vi "Measurement UI.vi"() -> ()   [LabVIEW 2021, in "audio_acMeasurement.lvlib"]
uses:
  audio_acMeasurement.lvlib
panel:
  in  "MeasGraphs":T1(tab)
  out "FreqDomainGraph":cluster{"x0":dbl, "dx":dbl, "magnitude":dbl[]}(graph) caption="AC"
  out "TimeDomainGraph":waveform(dbl)(graph) caption="AC"
  in  "JSON file":string
  out "Channel":string
  out "Spectrum":dbl[](array[numeric])
  out "df":dbl
  out "f0":dbl
  out "Time domain":dbl[](array[numeric])
  out "dt":dbl
  out "THD+N":dbl
  out "THD":dbl
  out "SNR":dbl
  out "Calculated amplitude":dbl
  out "Calculated frequency":dbl
  out "SFDR":dbl
  out "Dynamic range":dbl
  out "Gain error":dbl
  in  "Analog source resource name":string
  out "MeasTable":string[][](table)
  in  "File name":string(combo) caption="FILE NAME"
  out "Sample rate":u32 caption="SAMPLE RATE" format="%#.6pHz"
  in  "Protocol capture channel":string="0L" caption="CHANNEL"
  in  "Protocol capture resource name":string caption="RESOURCE NAME"
  in  "Protocol settings":string="Protocol settings"
  in  "Analog source":string="Analog source "
  in  "Full scale range":dbl=3.16 caption="FULL SCALE RANGE" format="%.3pV"
  in  "Measurement settings":string="Measurement settings"
  in  "MeasSettingsOptions":i32(listbox)=-1
  in  "MeasSettings":bool
  in  "DSGResourceName":tag caption="RESOURCE NAME"
  in  "Weighting filter":T2(ring) caption="WEIGHTING FILTER"
  in  "Number of words":u32=19200 caption="NUMBER OF WORDS"
  in  "Clock rate":u32=12288000 caption="CLOCK RATE" format="%#.6pHz"
  in  "Band stop":dbl=20000.0 caption="BAND STOP" format="%#_6pHz"
  in  "Band start":dbl=20.0 caption="BAND START" format="%#_6pHz"
  in  "Amplitude":dbl=-1.0 caption="AMPLITUDE" format="%#_6pdB"
  in  "Frequency":dbl=1000.0 caption="FREQUENCY" format="%#_6pHz"
  in  "Sensitivity":dbl=0.34762 caption="SENSITIVITY" format="%.5fFS/Pa"
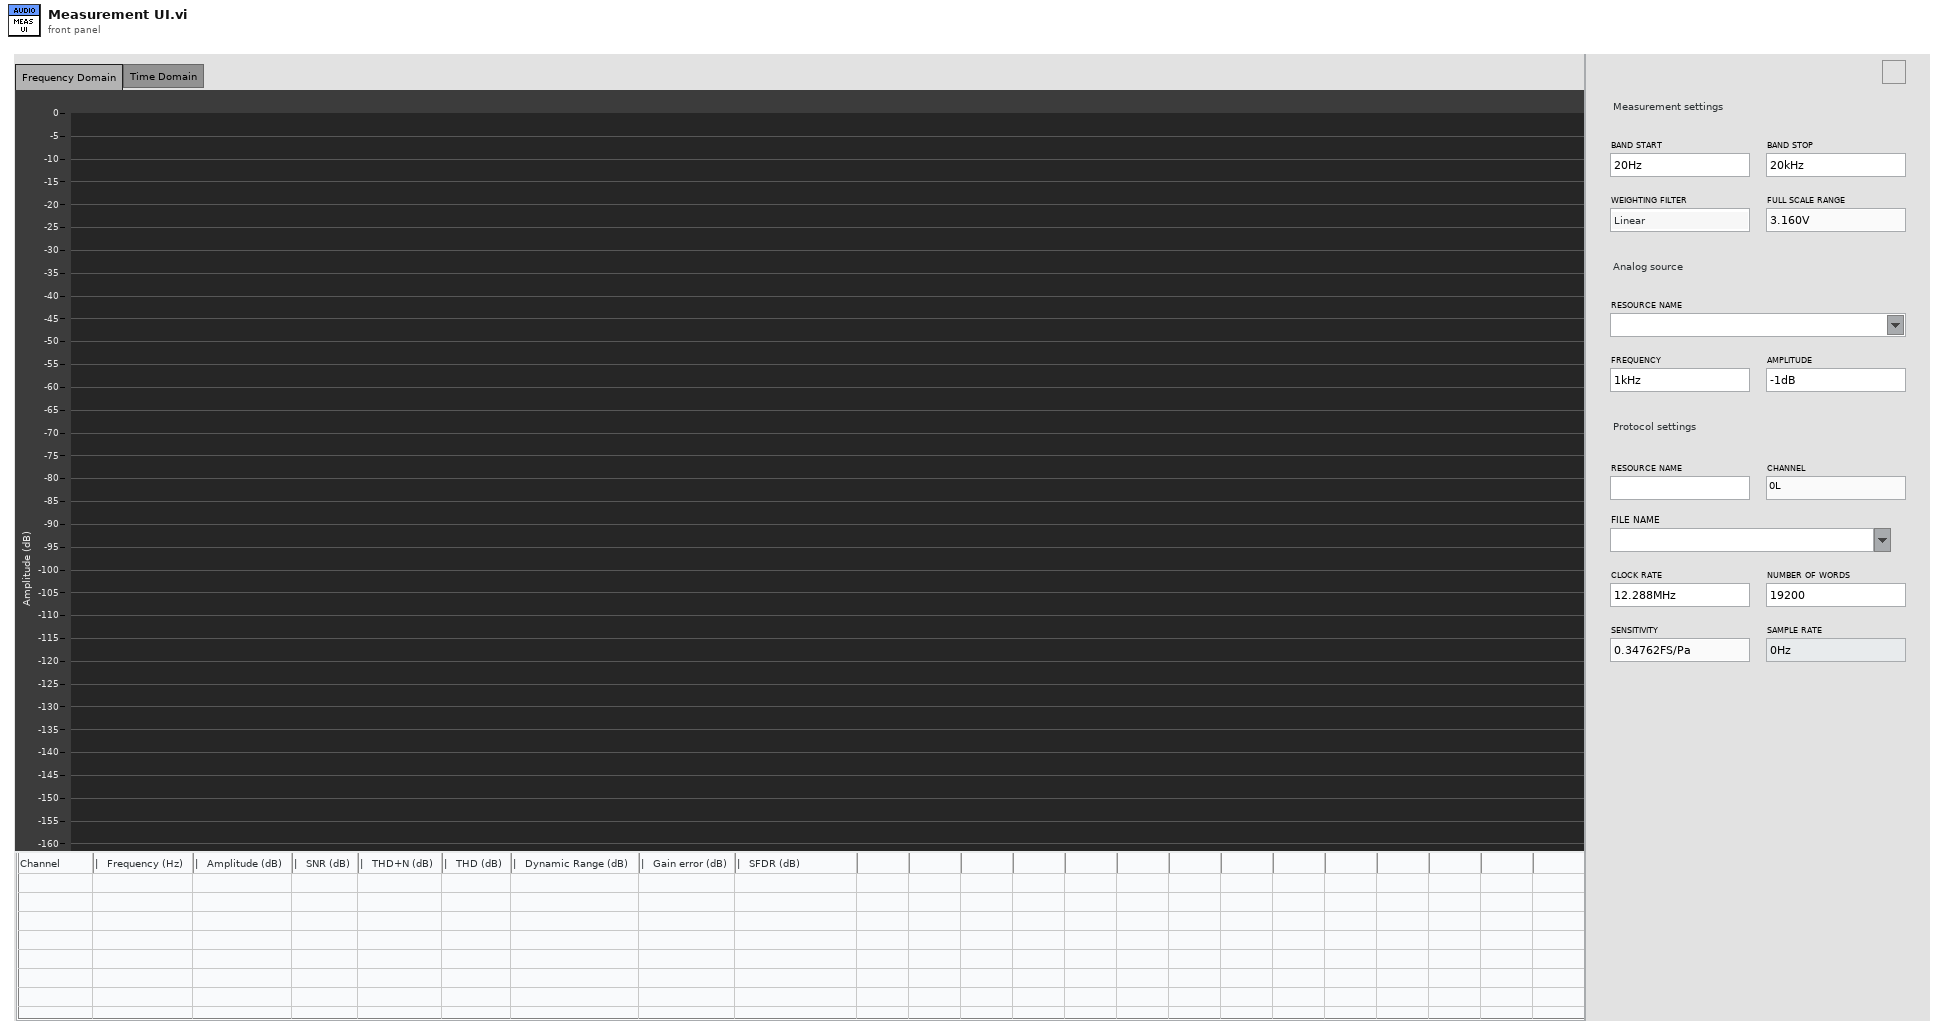
[diagram p1: front panel]
types:
  T1 = enum32{"Frequency Domain", "Time Domain", "Hidden Controls"}
  T2 = enum16{"Linear", "A-Weighting", "B-Weighting", "C-Weighting"}
  T3 = enum16{"open", "replace", "create", "open or create", "replace or create", "replace or create with confirmation"}
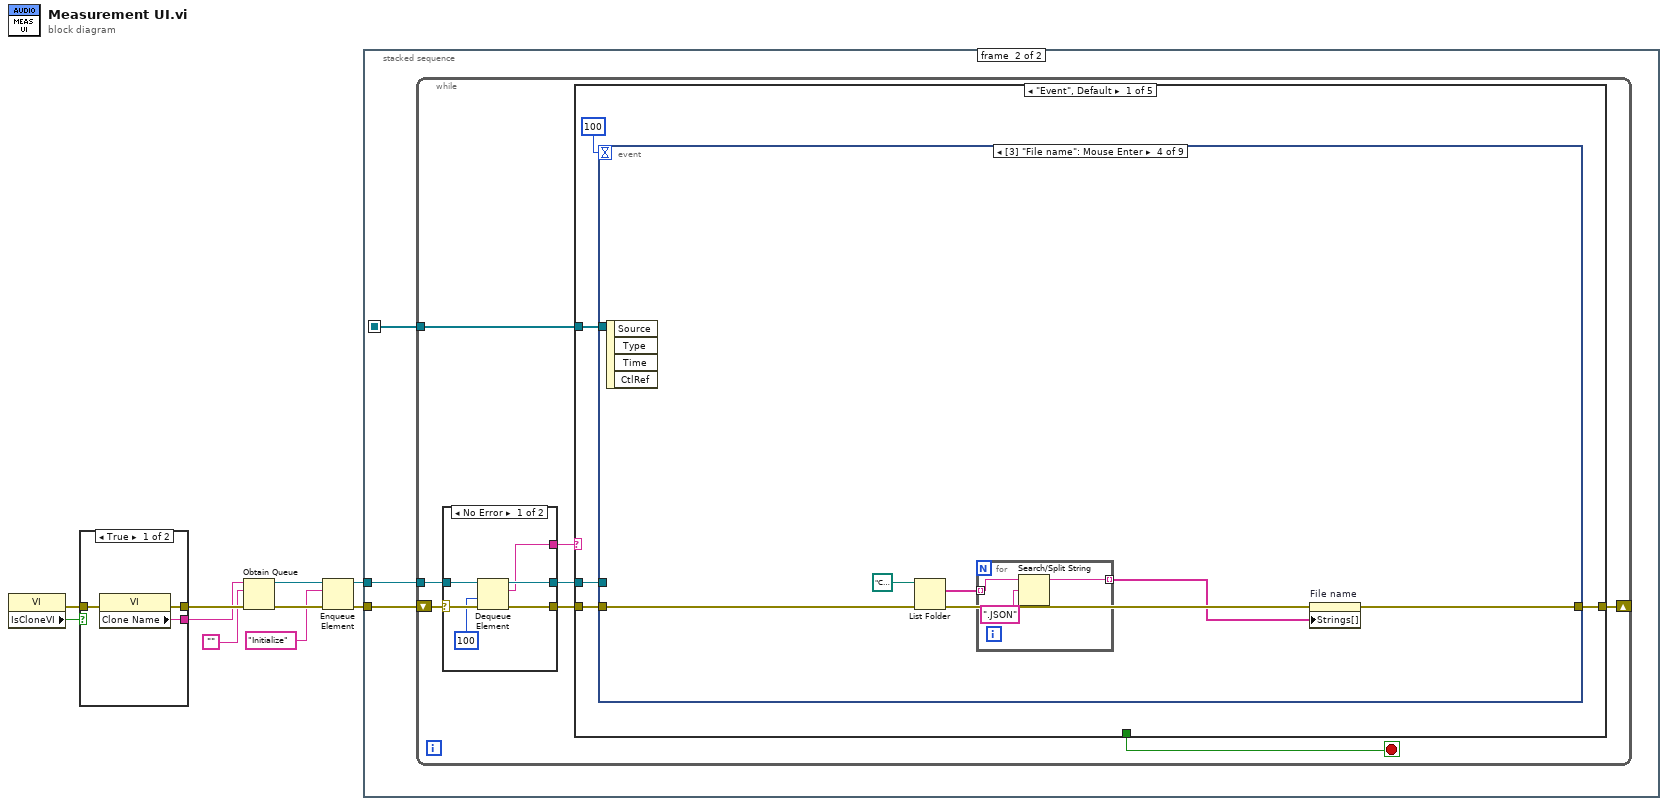
[diagram p0: block diagram]
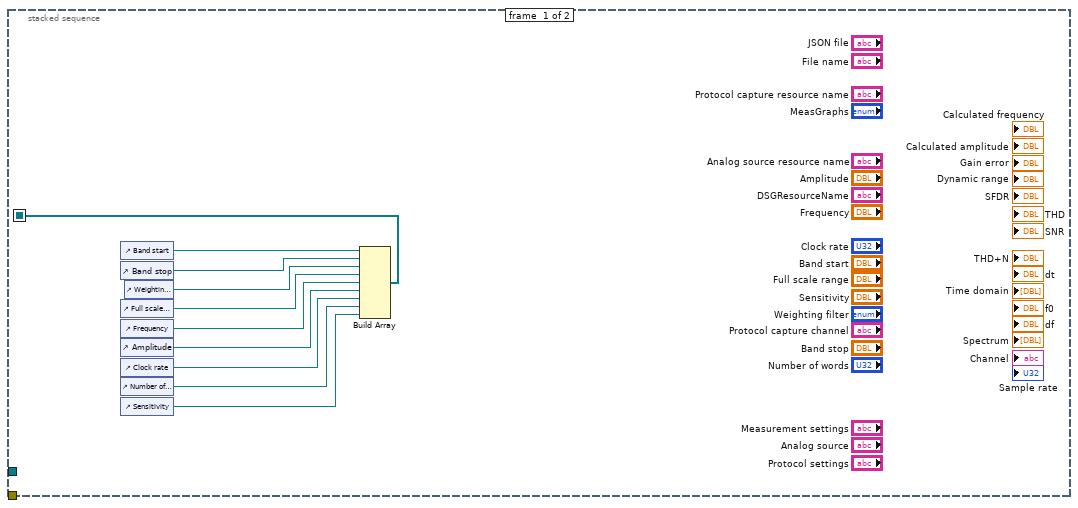
[diagram p2: hidden frame]
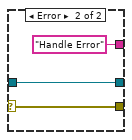
[diagram p3: hidden frame]
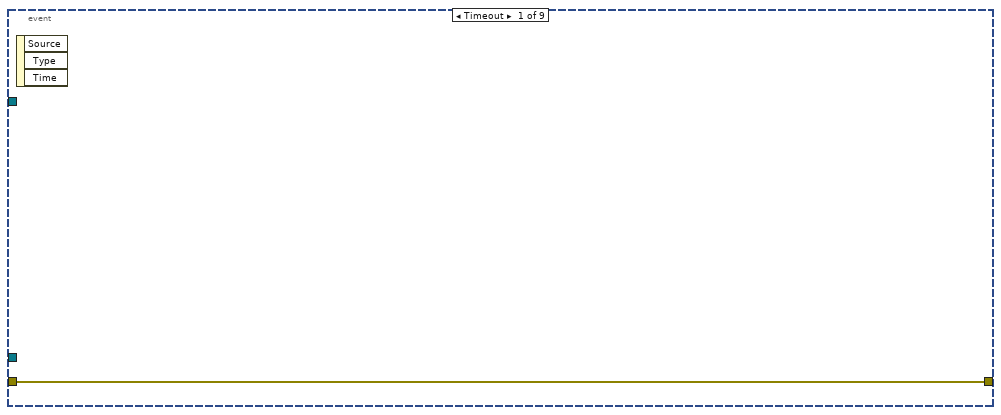
[diagram p4: hidden frame]
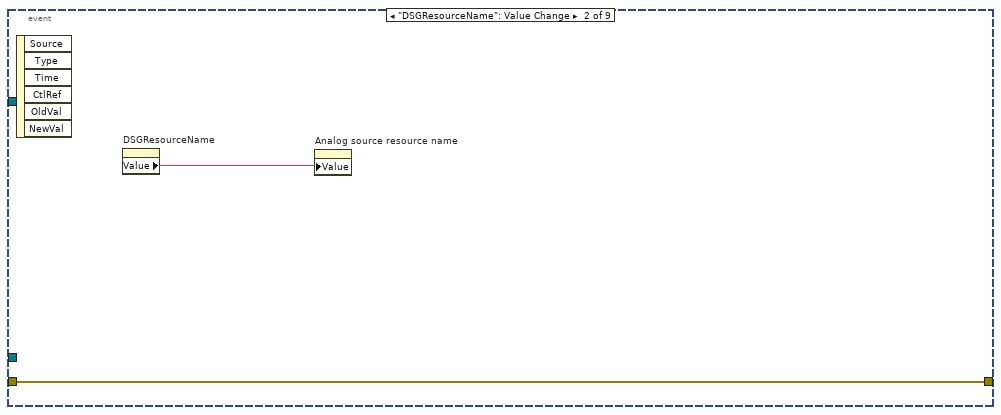
[diagram p5: hidden frame]
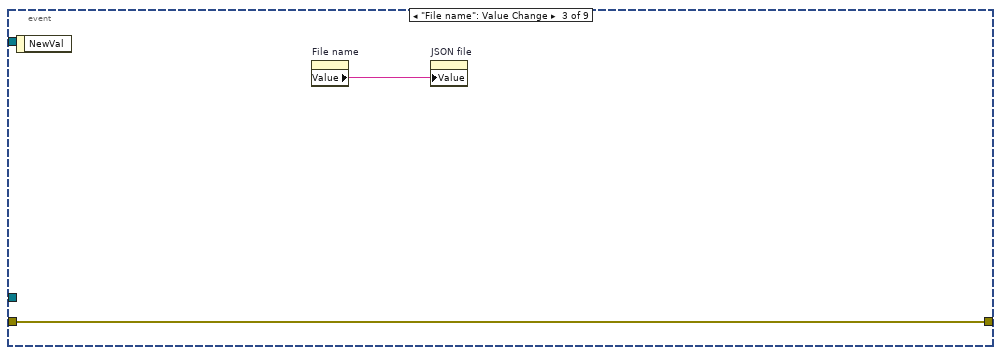
[diagram p6: hidden frame]
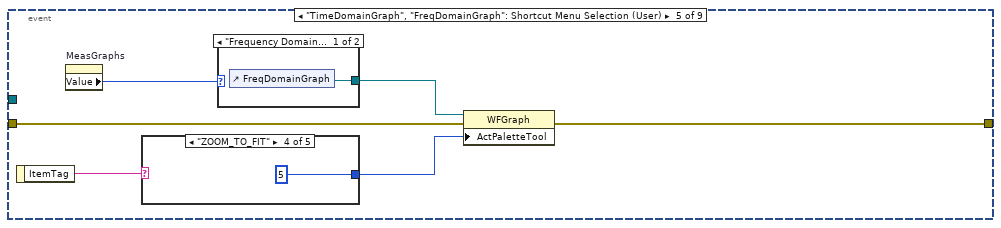
[diagram p7: hidden frame]
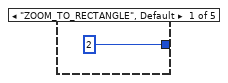
[diagram p8: hidden frame]
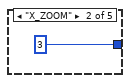
[diagram p9: hidden frame]
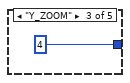
[diagram p10: hidden frame]
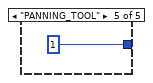
[diagram p11: hidden frame]
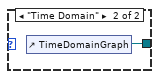
[diagram p12: hidden frame]
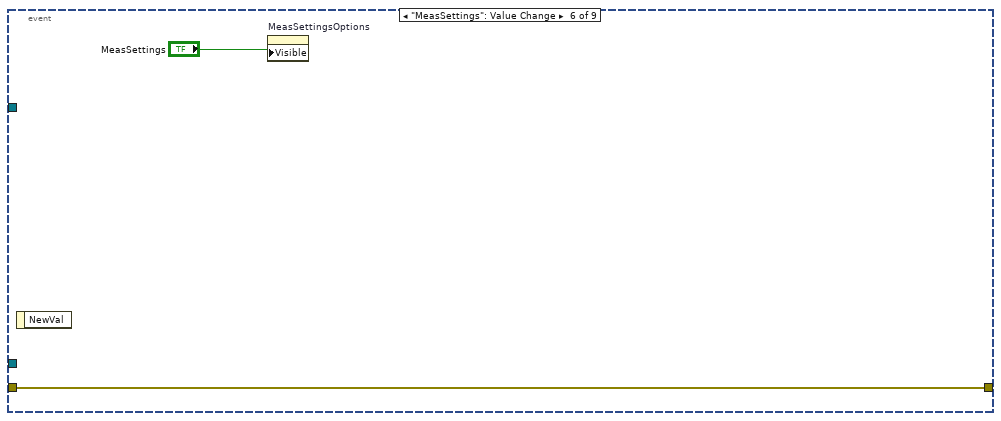
[diagram p13: hidden frame]
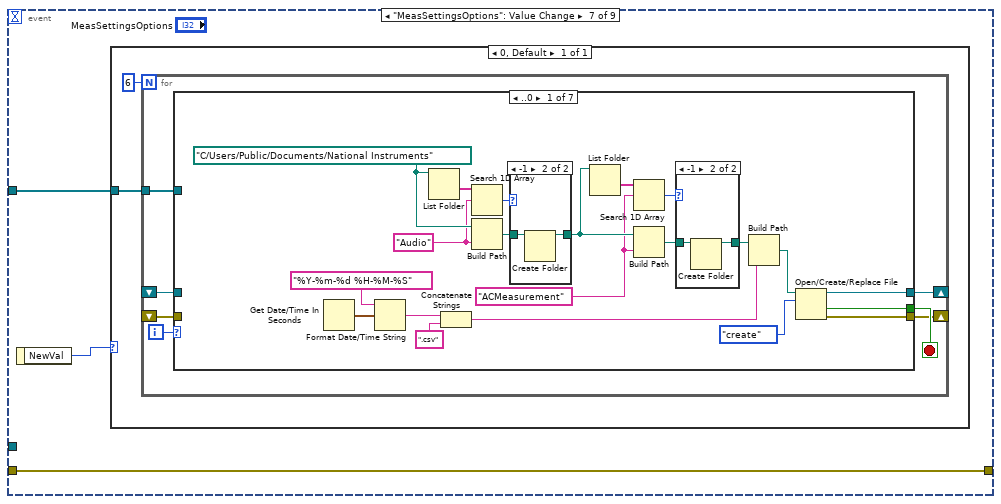
[diagram p14: hidden frame]
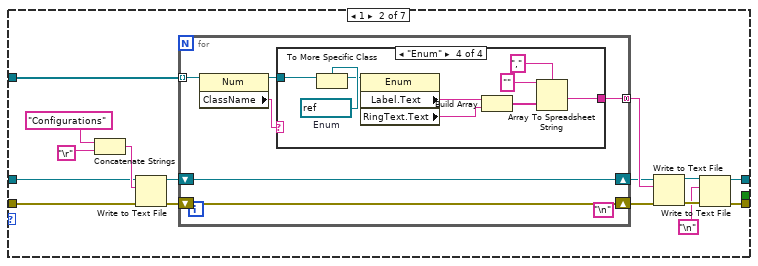
[diagram p17: hidden frame]
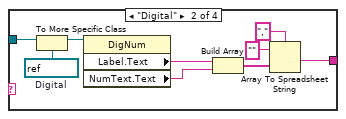
[diagram p19: hidden frame]
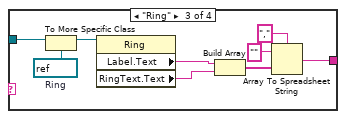
[diagram p20: hidden frame]
diagram:
  n1 = property class="VI"() -> (error out=w1:errorcluster, "IsCloneVI"=w2:bool)  [unwired: 2 in, 1 out]
  n2 = case shown="True" w2 {
    tunnel: [w13 w16] -> w10
    tunnel: [w12 w15] -> w9
    tunnel: w1 -> [w11 w14]
    frame True {
      n3 = property class="VI"(error in=w11) -> (error out=w13:errorcluster, "Clone Name"=w12:string)  [unwired: 1 in, 1 out]
    }
    frame False {
      n4 = property class="VI"(error in=w14) -> (error out=w16:errorcluster, "Name"=w15:string)  [unwired: 1 in, 1 out]
    }
  }
  n5 = Obtain Queue(name (unnamed)=w9, element data type="", error in (no error)=w10) -> (queue out=w6:refnum<queue>, error out=w8:errorcluster)  [unwired: 2 in, 1 out]
  n6 = Enqueue Element(queue=w6, element="Initialize", error in (no error)=w8) -> (queue out=w5:refnum<queue>, error out=w7:errorcluster)  [unwired: 1 in, 1 out]
  n7 = stacked-sequence {
    seq-local: [w23 _] -> [_ w27]
    tunnel: w7 -> [_ w29]
    tunnel: w5 -> [_ w28]
    frame #0 {
      n8 = control-ref of="Band start"() -> (w26:refnum<vi>)
      n9 = control-ref of="Band stop"() -> (w25:refnum<vi>)
      n10 = control-ref of="Full scale range"() -> (w22:refnum<vi>)
      n11 = control-ref of="Frequency"() -> (w21:refnum<vi>)
      n12 = control-ref of="Amplitude"() -> (w20:refnum<vi>)
      n13 = control-ref of="Clock rate"() -> (w19:refnum<vi>)
      n14 = control-ref of="Number of words"() -> (w18:refnum<vi>)
      n15 = control-ref of="Sensitivity"() -> (w17:refnum<vi>)
      n16 = control-ref of="Weighting filter"() -> (w24:refnum<vi>)
      n17 = Build Array(w26, w25, w24, w22, w21, w20, w19, w18, w17) -> (w23:refnum<vi>[])
    }
    frame #1 {
      n18 = while {
        shift-right: [w32] -> _
        shift-left: w29 -> [w37]
        tunnel: w28 -> [w35]
        tunnel: w27 -> [w30]
        stop <- w31 stop-if-true
        n19 = case shown="No Error" w37 {
          selector: w37 -> [w43 w46]
          tunnel: [w42 w46] -> w36
          tunnel: w35 -> [w41 w45]
          tunnel: [w40 w45] -> w34
          tunnel: [w39 "Handle Error"] -> w33
          frame No Error {
            n20 = Dequeue Element(queue=w41, timeout in ms (-1)=100, error in (no error)=w43) -> (queue out=w40:refnum<queue>, element=w39:string, error out=w42:errorcluster)  [unwired: 1 out]
          }
          frame Error {
          }
        }
        n21 = case shown="\"Event\", Default" w33 {
          tunnel: w36 -> [w50 w290 w328 w343 w344]
          tunnel: w34 -> [w48 _ _ w341 _]
          tunnel: [w51 w290 w328 w338 w344] -> w32
          tunnel: [_ _ _ TRUE _] -> w31
          tunnel: w30 -> [w47 _ _ _ _]
          frame "Event", Default {
            n22 = event shown="[3] \"File name\": Mouse Enter" {
              selector: _ -> [_ _ _ _ _ _ _ _ _]
              dyn-events: _ -> [_ _ _ _ _ _ _ _ _]
              timeout: 100 -> [_ _ _ _ _ _ _ _ _]
              tunnel: [w52 w53 w55 w58 w68 _ w83 w275 w280] -> w51
              tunnel: w50 -> [w52 w53 w55 w60 w67 w79 w83 w275 w281]
              tunnel: w48 -> [_ _ _ _ _ _ _ _ w279]
              tunnel: [_ _ _ _ _ w79 _ _ _] -> _
              tunnel: w47 -> [_ _ _ _ _ _ w81 _ _]
              event Timeout {
                n23 = event-data() -> ()  [unwired: 1 in, 3 out]
              }
              event "DSGResourceName": Value Change {
                n24 = event-data() -> ()  [unwired: 1 in, 6 out]
                n25 = property on="DSGResourceName" class="DAQmxName"() -> ("Value"=w54:string)  [unwired: 2 in, 2 out]
                n26 = property on="Analog source resource name" class="Str"("Value"=w54) -> ()  [unwired: 2 in, 2 out]
              }
              event "File name": Value Change {
                n27 = event-data() -> ()  [unwired: 1 in, 1 out]
                n28 = property on="File name" class="CmbBox"() -> ("Value"=w56:string)  [unwired: 2 in, 2 out]
                n29 = property on="JSON file" class="Str"("Value"=w56) -> ()  [unwired: 2 in, 2 out]
              }
              event "File name": Mouse Enter {
                n30 = event-data() -> ()  [unwired: 1 in, 4 out]
                n31 = List Folder(path=path "C:/Users/Public/Documents/National Instruments/Audio/Protocols", error in=w60) -> (filenames=w62:string[], error out=w59:errorcluster)  [unwired: 2 in, 2 out]
                n32 = for {
                  tunnel: w62 -> [w64] mode=indexing
                  tunnel: [w65] -> w57 mode=indexing
                  n33 = Search/Split String(string=w64, search string/char (-)=".JSON") -> (substring before match=w65:string)  [unwired: 1 in, 2 out]
                }
                n34 = property on="File name" class="CmbBox"(error in=w59, "Strings[]"=w57) -> (error out=w58:errorcluster)  [unwired: 1 in, 1 out]
              }
              event "TimeDomainGraph", "FreqDomainGraph": Shortcut Menu Selection (User) {
                n35 = event-data() -> ("ItemTag"=w70:string)  [unwired: 1 in]
                n36 = property on="MeasGraphs" class="TabCtl (strict)"() -> ("Value"=w71:T1)  [unwired: 2 in, 2 out]
                n37 = case shown="\"ZOOM_TO_FIT\"" w70 {
                  tunnel: [2 3 4 5 1] -> w66
                  frame "ZOOM_TO_RECTANGLE", Default {
                  }
                  frame "X_ZOOM" {
                  }
                  frame "Y_ZOOM" {
                  }
                  frame "ZOOM_TO_FIT" {
                  }
                  frame "PANNING_TOOL" {
                  }
                }
                n38 = case shown="\"Frequency Domain\", Default" w71 {
                  tunnel: [w77 w78] -> w69
                  frame "Frequency Domain", Default {
                    n39 = control-ref of="FreqDomainGraph"() -> (w77:refnum<vi>)
                  }
                  frame "Time Domain" {
                    n40 = control-ref of="TimeDomainGraph"() -> (w78:refnum<vi>)
                  }
                }
                n41 = property class="WFGraph"(reference=w69, error in=w67, "ActPaletteTool"=w66) -> (error out=w68:errorcluster)  [unwired: 1 out]
              }
              event "MeasSettings": Value Change {
                n42 = event-data() -> ()  [unwired: 1 in, 1 out]
                n43 = property on="MeasSettingsOptions" class="LstBox (strict)"("Visible"="MeasSettings") -> ()  [unwired: 2 in, 2 out]
              }
              event "MeasSettingsOptions": Value Change {
                n44 = event-data() -> ("NewVal"=w82:i32)  [unwired: 1 in]
                n45 = case shown="0, Default" w82 {
                  tunnel: w81 -> [w84]
                  frame 0, Default {
                    n46 = for {
                      N: 6 -> [_]
                      shift-right: [w90] -> _
                      shift-left: _ -> [w89]
                      shift-right: [w88] -> _
                      shift-left: _ -> [w87]
                      tunnel: w84 -> [w86]
                      i -> [w92]
                      stop <- w91 stop-if-true
                      n47 = case shown="..0" w92 {
                        tunnel: [w106 _ _ _ _ _ _] -> w91
                        tunnel: [w112 w132 w176 w203 w244 refnum<file> refnum ("refnum out") w274] -> w90
                        tunnel: w89 -> [_ w129 w187 w226 w245 w272 w274]
                        tunnel: [w105 w131 w175 w201 w243 w270 w273] -> w88
                        tunnel: w87 -> [_ w127 w186 w225 w246 w269 w273]
                        tunnel: w86 -> [_ w130 _ _ _ _ _]
                        frame ..0 {
                          w101 = "ACMeasurement" ("prompt")
                          w108 = "Audio" ("prompt")
                          w111 = path "C:/Users/Public/Documents/National Instruments" ("base path")
                          n48 = Get Date/Time In Seconds() -> (seconds since 1Jan1904=w98:timestamp)
                          n49 = Format Date/Time String(time format string (%c)="%Y-%m-%d %H-%M-%S", seconds (now)=w98) -> (date/time string=w97:string)  [unwired: 1 in]
                          n50 = List Folder(path=w111) -> (folder names=w109:string[])  [unwired: 3 in, 3 out]
                          n51 = Concatenate Strings(w97, ".csv" ("string")) -> (w94:string)
                          n52 = Search 1D Array(1D array=w109, element=w108) -> (index of element=w107:i32)  [unwired: 1 in]
                          n53 = Build Path(base path=w111, name or relative path=w108) -> (appended path=w110:path)
                          n54 = case shown="-1" w107 {
                            tunnel: w110 -> [w117 w119]
                            tunnel: [w117 w118] -> w102
                            frame Default {
                            }
                            frame -1 {
                              n55 = Create Folder(path (use dialog)=w119) -> (created path=w118:path)  [unwired: 2 in, 2 out]
                            }
                          }
                          n56 = List Folder(path=w102) -> (folder names=w104:string[])  [unwired: 3 in, 3 out]
                          n57 = Search 1D Array(1D array=w104, element=w101) -> (index of element=w103:i32)  [unwired: 1 in]
                          n58 = Build Path(base path=w102, name or relative path=w101) -> (appended path=w100:path)
                          n59 = case shown="-1" w103 {
                            tunnel: w100 -> [w114 w116]
                            tunnel: [w114 w115] -> w95
                            frame Default {
                            }
                            frame -1 {
                              n60 = Create Folder(path (use dialog)=w116) -> (created path=w115:path)  [unwired: 2 in, 2 out]
                            }
                          }
                          n61 = Build Path(base path=w95, name or relative path=w94) -> (appended path=w93:path)
                          n62 = Open/Create/Replace File(file path (use dialog)=w93, operation (0:open)=T3."create") -> (refnum out=w112:refnum<file>, cancelled=w106:bool, error out=w105:errorcluster)  [unwired: 4 in]
                        }
                        frame 1 {
                          (unwired) "\n"
                          n63 = Concatenate Strings("Configurations" ("format string"), "\r") -> (w133:string)
                          n64 = Write to Text File(file (use dialog)=w129, text=w133, error in=w127) -> (refnum out=w126:refnum<file>, error out=w128:errorcluster)  [unwired: 1 in, 1 out]
                          n65 = for {
                            tunnel: w130 -> [w137] mode=indexing
                            shift-right: [w141] -> w124
                            shift-left: w126 -> [w141]
                            shift-right: [w140] -> w123
                            shift-left: w128 -> [w140]
                            tunnel: [w139] -> w125 mode=concatenating
                            n66 = property class="Num"(reference=w137) -> (reference out=w138:refnum<vi>, "ClassName"=w136:string)  [unwired: 1 in, 1 out]
                            n67 = case shown="\"Enum\"" w136 {
                              tunnel: [_ w145 w155 w164] -> w139
                              tunnel: w138 -> [_ w143 w153 w168]
                              frame Default {
                              }
                              frame "Digital" {
                                w142 = refnum<vi> refnum  # Digital
                                n68 = To More Specific Class(target class=w142, reference=w143) -> (specific class reference=w144:refnum<vi>)  [unwired: 1 in, 1 out]
                                n69 = property class="DigNum"(reference=w144) -> ("Label.Text"=w150:string, "NumText.Text"=w149:string)  [unwired: 1 in, 2 out]
                                n70 = Build Array(w150, w149) -> (w146:string[])
                                n71 = Array To Spreadsheet String(delimiter (Tab)=",", array=w146, 3:"" ("format string")) -> (spreadsheet string=w145:string)
                              }
                              frame "Ring" {
                                w152 = refnum<vi> refnum  # Ring
                                n72 = To More Specific Class(target class=w152, reference=w153) -> (specific class reference=w154:refnum<vi>)  [unwired: 1 in, 1 out]
                                n73 = property class="Ring"(reference=w154) -> ("Label.Text"=w151:string, "RingText.Text"=w159:string)  [unwired: 1 in, 2 out]
                                n74 = Build Array(w151, w159) -> (w156:string[])
                                n75 = Array To Spreadsheet String(delimiter (Tab)=",", array=w156, 3:"" ("format string")) -> (spreadsheet string=w155:string)
                              }
                              frame "Enum" {
                                w167 = refnum<vi> refnum  # Enum
                                n76 = To More Specific Class(target class=w167, reference=w168) -> (specific class reference=w163:refnum<vi>)  [unwired: 1 in, 1 out]
                                n77 = property class="Enum"(reference=w163) -> ("Label.Text"=w162:string, "RingText.Text"=w161:string)  [unwired: 1 in, 2 out]
                                n78 = Build Array(w162, w161) -> (w160:string[])
                                n79 = Array To Spreadsheet String(delimiter (Tab)=",", array=w160, 3:"" ("format string")) -> (spreadsheet string=w164:string)
                              }
                            }
                          }
                          n80 = Write to Text File(file (use dialog)=w124, text=w125, error in=w123) -> (refnum out=w122:refnum<file>, error out=w121:errorcluster)  [unwired: 1 in, 1 out]
                          n81 = Write to Text File(file (use dialog)=w122, text="\n", error in=w121) -> (refnum out=w132:refnum<file>, error out=w131:errorcluster)  [unwired: 1 in, 1 out]
                        }
                        frame 2 {
                          n82 = property on="MeasTable" class="Tbl (strict)"() -> ("Column Headers[]"=w170:string[], "Value"=w169:string[][])  [unwired: 2 in, 2 out]
                          n83 = Build Array (concatenate)(w170, w169) -> (w184:string[][])
                          n84 = for {
                            tunnel: w184 -> [w189] mode=indexing
                            tunnel: [w188] -> w183 mode=indexing
                            n85 = for {
                              tunnel: w189 -> [w191] mode=indexing
                              tunnel: [w190] -> w188 mode=indexing
                              n86 = Match Pattern(string=w191, regular expression="|") -> (before substring=w195:string, after substring=w194:string, offset past match=w197:i32)  [unwired: 1 in, 1 out]
                              n87 = Less Than 0?(x=w197) -> (x < 0?=w196:bool)
                              n88 = Select(t=w195, s=w196, f=w194) -> (s? t:f=w193:string)
                              n89 = Match Pattern(string=w193, regular expression="[\\t\\n\\r\\s]*$") -> (before substring=w190:string)  [unwired: 1 in, 3 out]
                            }
                          }
                          n90 = Concatenate Strings("Results" ("element"), "\r") -> (w171:string)
                          n91 = Write to Text File(file (use dialog)=w187, text=w171, error in=w186) -> (refnum out=w185:refnum<file>, error out=w179:errorcluster)  [unwired: 1 in, 1 out]
                          n92 = Array To Spreadsheet String(delimiter (Tab)=",", array=w183, 3:"" ("format string")) -> (spreadsheet string=w180:string)
                          n93 = Write to Text File(file (use dialog)=w185, text=w180, error in=w179) -> (refnum out=w178:refnum<file>, error out=w177:errorcluster)  [unwired: 1 in, 1 out]
                          n94 = Write to Text File(file (use dialog)=w178, text="\n", error in=w177) -> (refnum out=w176:refnum<file>, error out=w175:errorcluster)  [unwired: 1 in, 1 out]
                        }
                        frame 3 {
                          n95 = property on="FreqDomainGraph" class="WFGraph (strict)"() -> ("Value"=w206:cluster{"x0":dbl, "dx":dbl, "magnitude":dbl[]})  [unwired: 2 in, 2 out]
                          n96 = Concatenate Strings("Frequency Domain" ("string"), "\r") -> (w223:string)
                          n97 = Build Array("Frequency (Hz)", "Amplitude (dB)") -> (w222:string[])
                          n98 = Write to Text File(file (use dialog)=w226, text=w223, error in=w225) -> (refnum out=w219:refnum<file>, error out=w218:errorcluster)  [unwired: 1 in, 1 out]
                          n99 = Unbundle By Name(w206) -> ("dx"=w210:dbl, "x0"=w211:dbl, "magnitude"=w209:dbl[])
                          n100 = Array To Spreadsheet String(delimiter (Tab)=",", array=w222, 3:"" ("format string")) -> (spreadsheet string=w217:string)
                          n101 = Write to Text File(file (use dialog)=w219, text=w217, error in=w218) -> (refnum out=w216:refnum<file>, error out=w215:errorcluster)  [unwired: 1 in, 1 out]
                          n102 = for {
                            tunnel: w209 -> [w230] mode=indexing
                            tunnel: w210 -> [w234]
                            tunnel: w211 -> [w232]
                            tunnel: [w227] -> w212 mode=indexing
                            i -> [w235]
                            n103 = Multiply(x=w235, y=w234) -> (x*y=w233:dbl)
                            n104 = Add(x=w233, y=w232) -> (x+y=w231:dbl)
                            n105 = Format Into String(w231) -> (resulting string=w228:string)  [unwired: 3 in, 1 out]
                            n106 = Format Into String(w230) -> (resulting string=w229:string)  [unwired: 3 in, 1 out]
                            n107 = Build Array(w228, w229) -> (w227:string[])
                          }
                          n108 = Array To Spreadsheet String(delimiter (Tab)=",", array=w212, 3:"" ("format string")) -> (spreadsheet string=w208:string)
                          n109 = Write to Text File(file (use dialog)=w216, text=w208, error in=w215) -> (refnum out=w205:refnum<file>, error out=w204:errorcluster)  [unwired: 1 in, 1 out]
                          n110 = Write to Text File(file (use dialog)=w205, text="\n", error in=w204) -> (refnum out=w203:refnum<file>, error out=w201:errorcluster)  [unwired: 1 in, 1 out]
                        }
                        frame 4 {
                          n111 = property on="TimeDomainGraph" class="WFGraph (strict)"() -> ("Value"=w242:waveform(dbl))  [unwired: 2 in, 2 out]
                          n112 = Concatenate Strings("Time Domain" ("string"), "\r") -> (w258:string)
                          n113 = Write to Text File(file (use dialog)=w245, text=w258, error in=w246) -> (refnum out=w255:refnum<file>, error out=w254:errorcluster)  [unwired: 1 in, 1 out]
                          n114 = Build Array("Time (s)", "Amplitude (V)") -> (w257:string[])
                          n115 = Unbundle By Name(w242) -> ("dt"=w240:dbl, "Y"=w241:dbl[])
                          n116 = Array To Spreadsheet String(delimiter (Tab)=",", array=w257, 3:"" ("format string")) -> (spreadsheet string=w253:string)
                          n117 = Write to Text File(file (use dialog)=w255, text=w253, error in=w254) -> (refnum out=w252:refnum<file>, error out=w251:errorcluster)  [unwired: 1 in, 1 out]
                          n118 = for {
                            tunnel: [w264] -> w248 mode=indexing
                            tunnel: w241 -> [w263] mode=indexing
                            tunnel: w240 -> [w261]
                            i -> [w262]
                            n119 = Multiply(x=w261, y=w262) -> (x*y=w260:dbl)
                            n120 = Format Into String(w260) -> (resulting string=w265:string)  [unwired: 3 in, 1 out]
                            n121 = Format Into String(w263) -> (resulting string=w266:string)  [unwired: 3 in, 1 out]
                            n122 = Build Array(w265, w266) -> (w264:string[])
                          }
                          n123 = Array To Spreadsheet String(delimiter (Tab)=",", array=w248, 3:"" ("format string")) -> (spreadsheet string=w247:string)
                          n124 = Write to Text File(file (use dialog)=w252, text=w247, error in=w251) -> (refnum out=w244:refnum<file>, error out=w243:errorcluster)  [unwired: 1 in, 1 out]
                        }
                        frame 5 {
                          w267 = FALSE ("Visible")
                          n125 = Close File(refnum=w272, error in=w269) -> (error out=w270:errorcluster)  [unwired: 1 out]
                          n126 = property on="MeasSettingsOptions" class="LstBox (strict)"("Visible"=w267, "Value"=-1 ("MeasSettingsOptions")) -> ()  [unwired: 2 in, 2 out]
                          n127 = property on="MeasSettings" class="Bool (strict)"("Value"=w267) -> ()  [unwired: 2 in, 2 out]
                        }
                        frame Default {
                        }
                      }
                    }
                  }
                }
              }
              event Mouse Down {
                w276 = FALSE ("Visible")
                n128 = event-data() -> ()  [unwired: 1 in, 1 out]
                n129 = property on="MeasSettingsOptions" class="LstBox (strict)"("Visible"=w276, "Value"=-1 ("MeasSettingsOptions")) -> ()  [unwired: 2 in, 2 out]
                n130 = property on="MeasSettings" class="Bool (strict)"("Value"=w276) -> ()  [unwired: 2 in, 2 out]
              }
              event Panel Close? {
                n131 = event-data() -> ()  [unwired: 1 in, 4 out]
                n132 = Enqueue Element(queue=w279, element="Exit", error in (no error)=w281) -> (error out=w280:errorcluster)  [unwired: 1 in, 2 out]
                n133 = event-data("Discard?"=TRUE) -> ()  [unwired: 1 in, 1 out]
              }
            }
          }
          frame "Initialize" {
            w288 = string[] ["Export data"] ("Item Names")
            w284 = "<Select Device>"
            n134 = for {
              N: 2 -> [_]
              i -> [w293]
              n135 = case shown="0, Default" w293 {
                tunnel: [w296 w297] -> w294
                frame 0, Default {
                  n136 = control-ref of="FreqDomainGraph"() -> (w296:refnum<vi>)
                }
                frame 1 {
                  n137 = control-ref of="TimeDomainGraph"() -> (w297:refnum<vi>)
                }
              }
              n138 = property class="WFGraph"(reference=w294, "ActPaletteTool"=2 ("Palette:Active Tool")) -> ()  [unwired: 1 in, 2 out]
            }
            n139 = property on="File name" class="CmbBox"("Value"="<Select File>") -> ()  [unwired: 2 in, 2 out]
            n140 = property on="DSGResourceName" class="DAQmxName"("Value"=w284) -> ()  [unwired: 2 in, 2 out]
            n141 = property on="Protocol capture resource name" class="Str"("Value"=w284) -> ()  [unwired: 2 in, 2 out]
            n142 = property on="MeasSettingsOptions" class="LstBox (strict)"("Item Names"=w288, "Value"=-1 ("MeasSettingsOptions"), "Visible"=FALSE, "Disabled Items"=i32[] []) -> ()  [unwired: 2 in, 2 out]
            n143 = for {
              tunnel: w288 -> [_] mode=indexing
              i -> [w292]
              n144 = property on="MeasSettingsOptions" class="LstBox (strict)"("Active Row"=w292, "Cell Height"=30 ("Active Row:Cell Height")) -> ()  [unwired: 2 in, 2 out]
            }
          }
          frame "Post UI Update" {
            w310 = "|   " ("initial string")
            # "This case will be triggered, after framework updates the User interface with result values."
            n145 = local read "Time domain"() -> (w327:dbl[])
            n146 = local read "Spectrum"() -> (w301:dbl[])
            n147 = local read "df"() -> (w303:dbl)
            n148 = local read "dt"() -> (w326:dbl)
            n149 = local read "f0"() -> (w300:dbl)
            n150 = local read "Calculated frequency"() -> (w313:dbl)
            n151 = local read "Calculated amplitude"() -> (w312:dbl)
            n152 = local read "Dynamic range"() -> (w322:dbl)
            n153 = Bundle By Name("Y"=w327, "dt"=w326) -> (→"TimeDomainGraph":waveform(dbl))  [unwired: 1 in]
            n154 = Bundle(cluster=cluster{"x0":dbl, "dx":dbl, "magnitude":dbl[]} {"x0"=0.0, "dx"=0.0, "magnitude"=[]} ("FreqDomainGraph"), "x0"=w300, "dx"=w303, "magnitude"=w301) -> (→"FreqDomainGraph":cluster{"x0":dbl, "dx":dbl, "magnitude":dbl[]})
            n155 = local read "THD+N"() -> (w323:dbl)
            n156 = local read "Gain error"() -> (w309:dbl)
            n157 = local read "THD"() -> (w324:dbl)
            n158 = local read "SNR"() -> (w311:dbl)
            n159 = local read "SFDR"() -> (w308:dbl)
            n160 = Build Array(w313, w312) -> (w319:dbl[])
            n161 = Build Array(w311, w323, w324, w322) -> (w318:dbl[])
            n162 = for {
              tunnel: w319 -> [w333] mode=indexing
              tunnel: w310 -> [w334]
              tunnel: "%.3f" ("initial string") -> [w335]
              tunnel: [w336] -> w317 mode=indexing
              n163 = Format Into String(format string=w335, initial string=w334, w333) -> (resulting string=w336:string)  [unwired: 1 in, 1 out]
            }
            n164 = for {
              tunnel: w318 -> [w329] mode=indexing
              tunnel: w310 -> [w330]
              tunnel: "%5.1f" ("initial string") -> [w331]
              tunnel: [w332] -> w316 mode=indexing
              n165 = Format Into String(format string=w331, initial string=w330, w329) -> (resulting string=w332:string)  [unwired: 1 in, 1 out]
            }
            n166 = Format Into String(format string="%5.1f" ("initial string"), initial string=w310, w308) -> (resulting string=w306:string)  [unwired: 1 in, 1 out]
            n167 = Format Into String(format string="%5.3f" ("initial string"), initial string=w310, w309) -> (resulting string=w307:string)  [unwired: 1 in, 1 out]
            n168 = local read "Channel"() -> (w298:string)
            n169 = Build Array (concatenate)(w298, w317, w316, w307, w306) -> (w315:string[])
            n170 = Build Array(w315) -> (→"MeasTable":string[][])
          }
          frame "Exit" {
            # "This case is triggered to close the User Interface from framework"
            n171 = Flush Queue(queue=w341, error in (no error)=w343) -> (queue out=w340:refnum<queue>, error out=w339:errorcluster)  [unwired: 1 out]
            n172 = Release Queue(queue=w340, force destroy? (F)=TRUE, error in (no error)=w339) -> (error out=w338:errorcluster)  [unwired: 2 out]
          }
          frame "Handle Error" {
          }
        }
      }
    }
  }
